vi "Get Colors.vi"(11 "Blue Plugin in":refnum<class "Blue Plugin.lvclass">) -> (3 "Color Box":u32(colorbox))   [LabVIEW 2020, in "Blue Plugin.lvclass"]
uses:
  Blue Plugin.lvclass
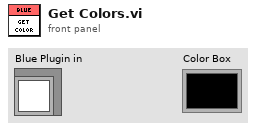
[diagram p1: front panel]
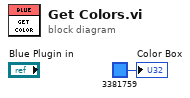
[diagram p0: block diagram]
diagram:
  "Color Box" <- u32 3381759 ("Color Box")
